vi "Read Acquisition Complete.vi"(8 "error in (no error)":errorcluster, 11 "Scope Instrument in":refnum<class "Scope Instrument.lvclass">) -> (0 "error out":errorcluster, 2 "Acquisition Complete":bool, 3 "Scope Instrument out":refnum<class "Scope Instrument.lvclass">)   [LabVIEW 2025, in "Scope.lvlib" / "Scope Instrument.lvclass"]
uses:
  Scope Instrument.lvclass
  Scope Instrument.lvclass/Scope Instrument.ctl
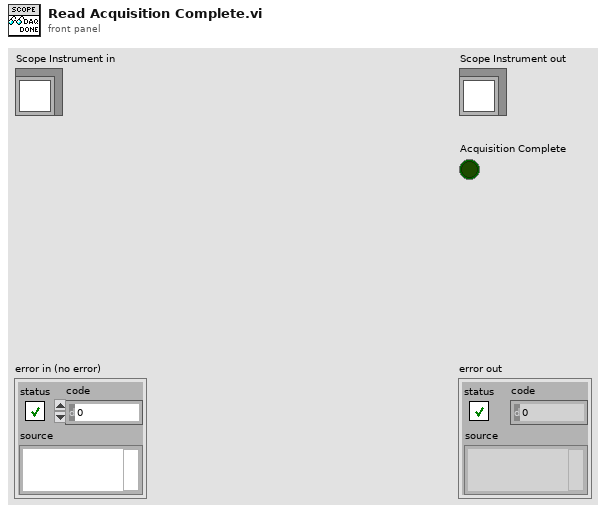
[diagram p1: front panel]
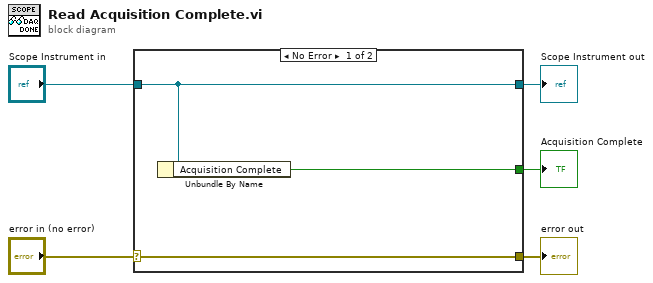
[diagram p0: block diagram]
diagram:
  n1 = case shown="No Error" "error in (no error)" {
    selector: "error in (no error)" -> [w8 w9]
    tunnel: [w8 w9] -> w4
    tunnel: [w7 w10] -> w2
    tunnel: "Scope Instrument in" -> [w7 w10]
    tunnel: [w6 _] -> w1
    frame No Error {
      n2 = Unbundle By Name(w7) -> ("Acquisition Complete"=w6:bool)
    }
    frame Error {
    }
  }
  "error out" <- w4
  "Scope Instrument out" <- w2
  "Acquisition Complete" <- w1
